vi "5a - DSTP write.vi"() -> ()   [LabVIEW 2010]
panel:
  out "cosx":dbl
  in  "stop":bool
  out "Chart":dbl(graph)
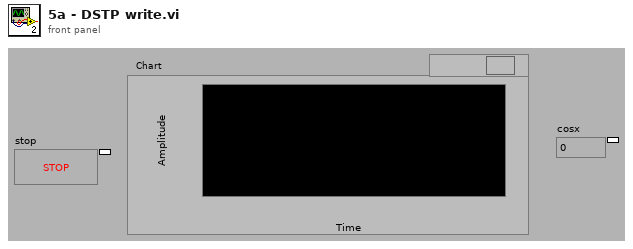
[diagram p1: front panel]
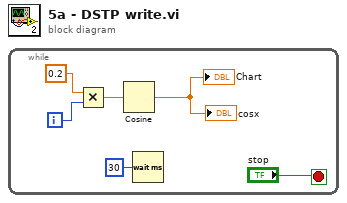
[diagram p0: block diagram]
diagram:
  n1 = while {
    i -> [w3]
    stop <- "stop" stop-if-true
    n2 = Multiply(x=0.2, y=w3) -> (x*y=w2:dbl)
    n3 = Cosine(x=w2) -> (cos(x)=→"Chart" →"cosx":dbl)
    n4 = Wait (ms)(milliseconds to wait=u32 30) -> ()  [unwired: 1 out]
  }
